vi "DDE Close Conversation.vi"(8 "error in (no error)":errorcluster, 10 "mode(T,close immediately)":bool, 11 "conversation refnum":u32) -> (0 "error out":errorcluster)   [LabVIEW 2018]
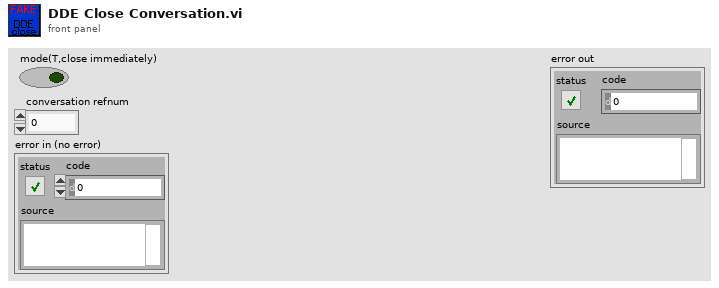
[diagram p1: front panel]
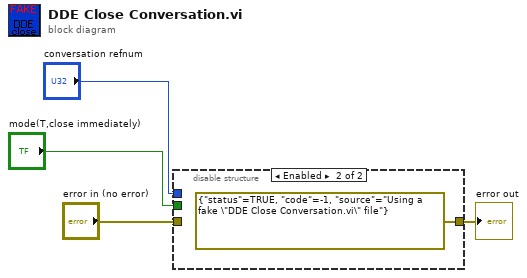
[diagram p0: block diagram]
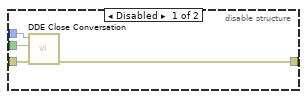
[diagram p2: hidden frame]
diagram:
  n1 = disable-structure shown="Enabled" {
    disable-tunnel: "conversation refnum" -> [w8 _]
    disable-tunnel: "error in (no error)" -> [w7 _]
    disable-tunnel: "mode(T,close immediately)" -> [w6 _]
    disable-tunnel: [w5 errorcluster {"status"=TRUE, "code"=-1, "source"="Using a fake \"DDE Close Conversation.vi\" file"} ("error out")] -> w1
    frame Disabled {
      n2 = call "DDE Close Conversation.vi"("error in (no error)"=w7, "mode(T,close immediately)"=w6, "conversation refnum"=w8) -> ("error out"=w5:errorcluster)  [unwired: 6 in]
    }
    frame Enabled {
    }
  }
  "error out" <- w1
